vi "이벤트 (열거형).vi"() -> ()   [LabVIEW 2014]
uses:
  <vilib>/Analysis/1siggen.llb/General Aperiodic Triangle.vi
  <vilib>/Analysis/NI_AALBase.lvlib
panel:
  out "웨이브폼 그래프":dbl[](graph)
  in  "정지":bool
  in  "열거형":enum16{"초기화", "Idle", "정지", "Task1", "Task2"}(ring)
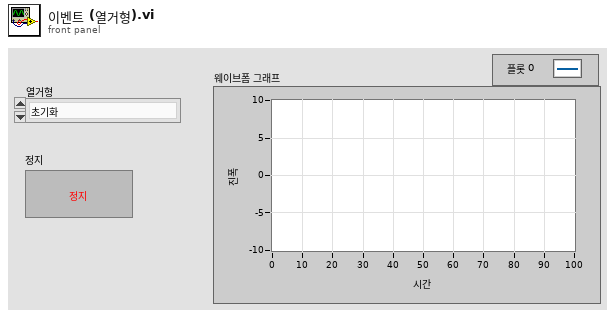
[diagram p1: front panel]
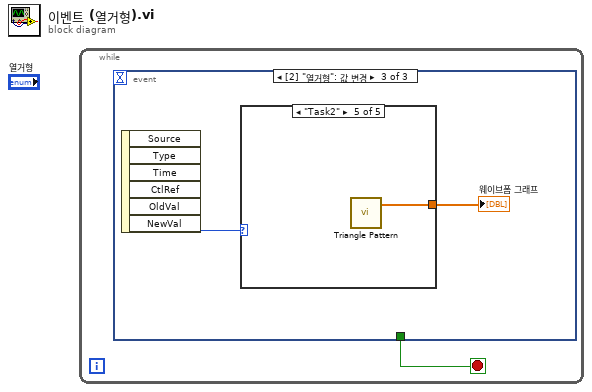
[diagram p0: block diagram]
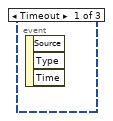
[diagram p2: hidden frame]
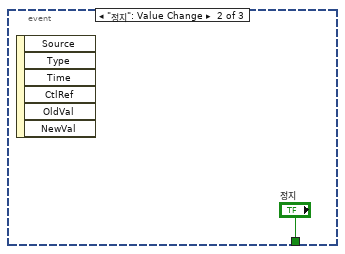
[diagram p3: hidden frame]
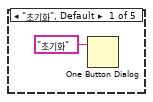
[diagram p4: hidden frame]
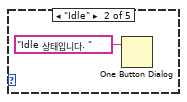
[diagram p5: hidden frame]
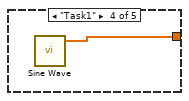
[diagram p7: hidden frame]
diagram:
  n1 = while {
    stop <- w1 stop-if-true
    n2 = event shown="[2] \"열거형\": 값 변경" {
      selector: _ -> [_ _ _]
      dyn-events: _ -> [_ _ _]
      timeout: _ -> [_ _ _]
      tunnel: [_ "정지" _] -> w1
      event Timeout {
        n3 = event-data() -> ()  [unwired: 1 in, 3 out]
      }
      event "정지": Value Change {
        n4 = event-data() -> ()  [unwired: 1 in, 6 out]
      }
      event "열거형": Value Change {
        n5 = event-data() -> ("NewVal"=w4:enum16{"초기화", "Idle", "정지", "Task1", "Task2"})  [unwired: 1 in, 5 out]
        n6 = case shown="\"Task2\"" w4 {
          tunnel: [_ _ _ w7 w8] -> w3
          frame "초기화", Default {
            n7 = One Button Dialog(message="초기화" ("메시지")) -> ()  [unwired: 1 in, 1 out]
          }
          frame "Idle" {
            n8 = One Button Dialog(message="Idle 상태입니다. " ("메시지")) -> ()  [unwired: 1 in, 1 out]
          }
          frame "정지" {
          }
          frame "Task1" {
            n9 = call <vilib>:"Sine Wave.vi"() -> ("sine wave"=w7:dbl[])  [unwired: 5 in, 2 out]
          }
          frame "Task2" {
            n10 = call <vilib>:"Triangle Pattern.vi"() -> ("Triangle Pattern"=w8:dbl[])  [unwired: 10 in, 1 out]
          }
        }
        "웨이브폼 그래프" <- w3
      }
    }
  }
